vi "GEOM_wcs_override_directive_parser.vi"(10 "modif in":string) -> (1 "override?":bool, 2 "modif out":string, 3 "last col":string)   [LabVIEW 2016]
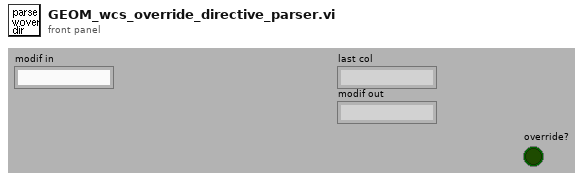
[diagram p1: front panel]
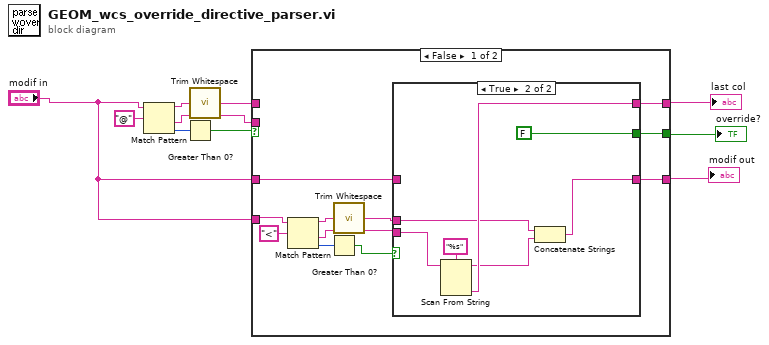
[diagram p0: block diagram]
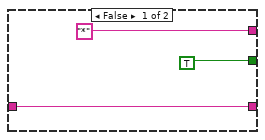
[diagram p2: hidden frame]
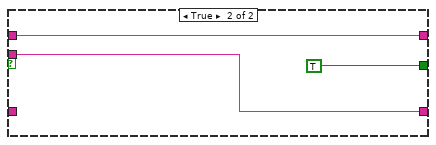
[diagram p3: hidden frame]
diagram:
  n1 = Match Pattern(string="modif in", regular expression="@") -> (before substring=w10:string, after substring=w3:string, offset past match=w9:i32)  [unwired: 2 out]
  n2 = Greater Than 0?(x=w9) -> (x > 0?=w7:bool)
  n3 = call <vilib>:"Trim Whitespace.vi"("string"=w10) -> ("trimmed string"=w6:string)  [unwired: 1 in]
  n4 = case shown="False" w7 {
    tunnel: w6 -> [_ w34]
    tunnel: [w21 w34] -> w5
    tunnel: "modif in" -> [w14 _]
    tunnel: [w13 w33] -> w4
    tunnel: w3 -> [_ w33]
    tunnel: [w15 TRUE ("override?")] -> w2
    tunnel: "modif in" -> [w17 _]
    frame False {
      n5 = Match Pattern(string=w17, regular expression="<") -> (before substring=w20:string, after substring=w11:string, offset past match=w19:i32)  [unwired: 2 out]
      n6 = Greater Than 0?(x=w19) -> (x > 0?=w16:bool)
      n7 = call <vilib>:"Trim Whitespace.vi"("string"=w20) -> ("trimmed string"=w12:string)  [unwired: 1 in]
      n8 = case shown="True" w16 {
        tunnel: ["*" ("f") w29] -> w21
        tunnel: [TRUE ("override?") FALSE ("override?")] -> w15
        tunnel: w14 -> [w22 _]
        tunnel: [w22 w26] -> w13
        tunnel: w12 -> [_ w25]
        tunnel: w11 -> [_ w28]
        frame False {
        }
        frame True {
          n9 = Scan From String(format string="%s", input string=w28) -> (remaining string=w27:string, output 1=w29:string)  [unwired: 2 in, 3 out]
          n10 = Concatenate Strings(w25, w27) -> (w26:string)
        }
      }
    }
    frame True {
    }
  }
  "last col" <- w5
  "modif out" <- w4
  "override?" <- w2
